vi "ErrorMessageBuilder.vi"(1 "Errors":T1(array[cluster]), 2 "Reset Error History":bool) -> (0 "Combined Error String":string)   [LabVIEW 2023]
doc: "This VI is used to convert a set of boolean triggers into an error message string which may be displayed or spoken aloud. The error messages will repeat with a period set by \"Delays.\""
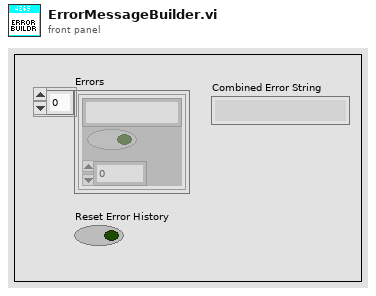
[diagram p1: front panel]
types:
  T1 = cluster{"Error Message":string, "Trigger":bool, "Delay (s)":dbl}[]
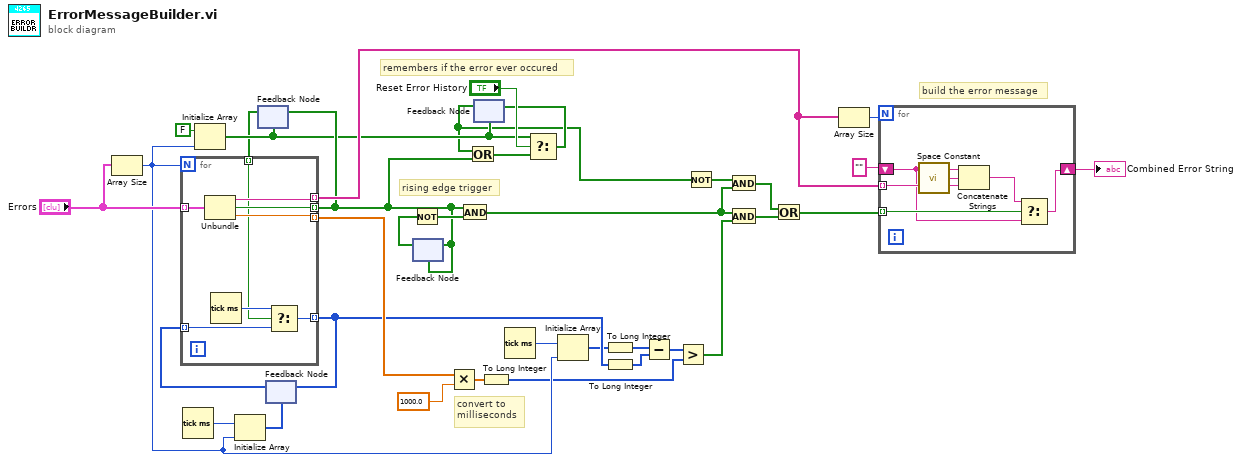
[diagram p0: block diagram]
diagram:
  # "convert to\nmilliseconds"
  # "remembers if the error ever occured"
  # "build the error message"
  # "rising edge trigger"
  n1 = Array Size(array="Errors") -> (size(s)=w14:i32)
  n2 = Tick Count (ms)() -> (millisecond timer value=w25:u32)
  n3 = Initialize Array(FALSE, w14) -> (w12:bool[])
  n4 = Initialize Array(w25, w14) -> (w24:u32[])
  n5 = feedback #1(w12) -> (w11:bool[])
  n6 = feedback #2(w24) -> (w28:u32[])
  n7 = for {
    N: w14 -> [_]
    tunnel: "Errors" -> [w43] mode=indexing
    tunnel: [w39] -> w15 mode=indexing
    tunnel: [w42] -> w31 mode=indexing
    tunnel: [w41] -> w30 mode=indexing
    tunnel: [w38] -> w23 mode=indexing
    tunnel: w28 -> [w37] mode=indexing
    tunnel: w11 -> [w36] mode=indexing
    n8 = Unbundle(w43) -> ("Error Message"=w42:string, "Trigger"=w39:bool, "Delay (s)"=w41:dbl)
    n9 = Tick Count (ms)() -> (millisecond timer value=w40:u32)
    n10 = Select(t=w40, s=w36, f=w37) -> (s? t:f=w38:u32)
  }
  n11 = feedback-in #1(w15) -> ()
  n12 = feedback-in #2(w23) -> ()
  n13 = feedback #3(w15) -> (w29:bool[])
  n14 = Not(x=w29) -> (.not. x?=w35:bool[])
  n15 = feedback-in #3(w15) -> ()
  n16 = Multiply(x=w30, y=1000.0) -> (x*y=w9:dbl[])
  n17 = And(x=w15, y=w35) -> (x .and. y?=w17:bool[])
  n18 = feedback #4(w12) -> (w1:bool[])
  n19 = Or(x=w1, y=w15) -> (x .or. y?=w21:bool[])
  n20 = To Long Integer(number=w9) -> (32bit integer=w10:i32[])
  n21 = Tick Count (ms)() -> (millisecond timer value=w7:u32)
  n22 = Select(t=w12, s="Reset Error History", f=w21) -> (s? t:f=w19:bool[])
  n23 = feedback-in #4(w19) -> ()
  n24 = Initialize Array(w7, w14) -> (w6:u32[])
  n25 = To Long Integer(number=w6) -> (32bit integer=w4:i32[])
  n26 = To Long Integer(number=w23) -> (32bit integer=w3:i32[])
  n27 = Subtract(x=w4, y=w3) -> (x-y=w5:i32[])
  n28 = Greater?(x=w5, y=w10) -> (0:w22:bool[])
  n29 = Not(x=w1) -> (.not. x?=w18:bool[])
  n30 = And(x=w18, y=w17) -> (x .and. y?=w16:bool[])
  n31 = And(x=w17, y=w22) -> (x .and. y?=w27:bool[])
  n32 = Or(x=w16, y=w27) -> (x .or. y?=w2:bool[])
  n33 = Array Size(array=w31) -> (size(s)=w32:i32)
  n34 = for {
    N: w32 -> [_]
    tunnel: w2 -> [w49] mode=indexing
    tunnel: w31 -> [w47] mode=indexing
    shift-right: [w45] -> w33
    shift-left: "" -> [w44]
    n35 = call <vilib>:"Space Constant.vi"() -> ("String"=w48:string)
    n36 = Concatenate Strings(w44, w48, w47) -> (w46:string)
    n37 = Select(t=w46, s=w49, f=w44) -> (s? t:f=w45:string)
  }
  "Combined Error String" <- w33
